vi "Shooter - Calculate Distance (SubVI).vi"(11 "offsetAngle V":dbl) -> (3 "Distance (inches)":dbl)   [LabVIEW 2019]
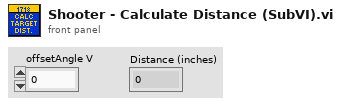
[diagram p1: front panel]
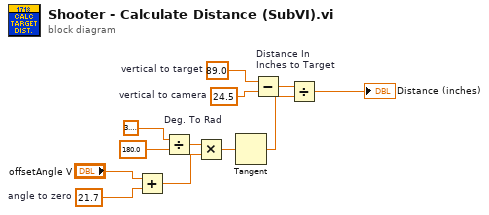
[diagram p0: block diagram]
diagram:
  w3 = 21.7  # angle to zero
  w1 = 24.5  # vertical to camera
  w2 = 89.0  # vertical to target
  n1 = Add(x="offsetAngle V", y=w3) -> (x+y=w4:dbl)
  n2 = Divide "Deg. To Rad"(x=3.141592653589793, y=180.0 ("x")) -> (x/y=w7:dbl)
  n3 = Multiply(x=w7, y=w4) -> (x*y=w8:dbl)
  n4 = Tangent(1:w8) -> (0:w9:dbl)
  n5 = Subtract(x=w2, y=w1) -> (x-y=w10:dbl)
  n6 = Divide "Distance In\nInches to Target"(x=w10, y=w9) -> (x/y=→"Distance (inches)":dbl)
